vi "sv_Build Frame for Octave.vi"(2 "Y maximum":dbl format="%.2f", 3 "X maximum":dbl format="%.2f", 4 "z scale":cluster{"z min":dbl, "z max":dbl} {"z max" format="%.2f"; "z min" format="%.2f"}, 5 "x scale":cluster{"x min":dbl, "x max":dbl} {"x max" format="%.2f"; "x min" format="%.2f"}) -> (0 "back frame":cluster{dbl[], dbl[]} {"?" format="%.2f"; "?" format="%.2f"}, 1 "front frame":cluster{dbl[], dbl[]} {"?" format="%.2f"; "?" format="%.2f"})   [LabVIEW 2017]
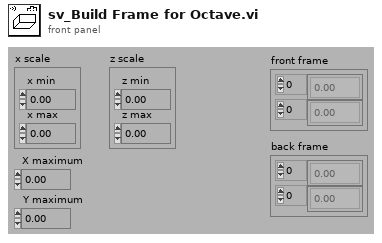
[diagram p1: front panel]
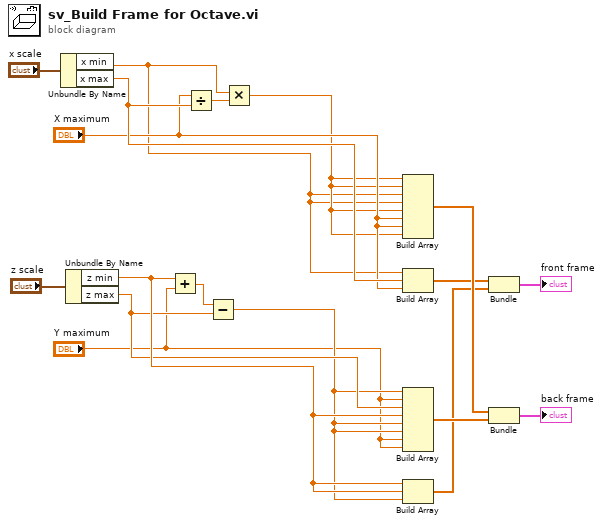
[diagram p0: block diagram]
diagram:
  n1 = Unbundle By Name("x scale") -> ("x min"=w1:dbl, "x max"=w5:dbl)
  n2 = Unbundle By Name("z scale") -> ("z min"=w9:dbl, "z max"=w8:dbl)
  n3 = Add(x=w9, y="Y maximum") -> (x+y=w18:dbl)
  n4 = Divide(x="X maximum", y=w5) -> (x/y=w2:dbl)
  n5 = Subtract(x=w18, y=w8) -> (x-y=w7:dbl)
  n6 = Multiply(x=w1, y=w2) -> (x*y=w3:dbl)
  n7 = Build Array(w3, w3, w1, w1, w3, "X maximum", "X maximum", w3) -> (w17:dbl[])
  n8 = Build Array(w1, w5, "X maximum") -> (w14:dbl[])
  n9 = Build Array(w7, "Y maximum", w8, w9, w7, w7, "Y maximum", "Y maximum") -> (w16:dbl[])
  n10 = Build Array(w9, w9, w7) -> (w13:dbl[])
  n11 = Bundle(w14, w13) -> (→"front frame":cluster{dbl[], dbl[]})  [unwired: 1 in]
  n12 = Bundle(w17, w16) -> (→"back frame":cluster{dbl[], dbl[]})  [unwired: 1 in]
